vi "Tell Child.vi"(4 "Priority":bool, 6 "UID":string, 7 "Actor in":refnum<class "Actor.lvclass">, 9 "Error":errorcluster, 10 "Actor":refnum<class "Actor.lvclass">) -> (0 "Error out":errorcluster)   [LabVIEW 2025, in "jettl.lvlib" / "Stopped jettl Msg.lvlib"]
uses:
  Stopped jettl Msg.lvlib
  Actor/Actor.lvclass
  Msg Input/Msg Input.lvclass
  Stopped Msg/Stopped Msg/Stopped Msg.lvclass
  C:/git/jettl/src/jettl/jettl/Stopped jettl Msg/Stopped Msg/Stopped Msg/Stopped Msg.lvclass
  C:/git/jettl/src/jettl/jettl/Msg/Msg.lvclass
  jettl.lvlib
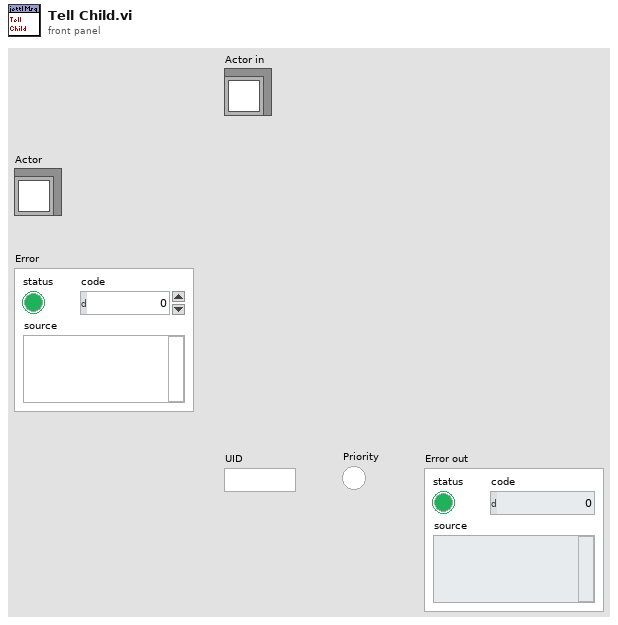
[diagram p1: front panel]
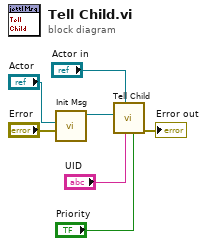
[diagram p0: block diagram]
diagram:
  n1 = call "Init Msg.vi"(9:"Error", "Msg Input"="Actor") -> ("Stopped Msg out"=w4:refnum<class "Stopped Msg.lvclass">)  [unwired: 9 in]
  n2 = call "Tell Child.vi"("Priority"="Priority", "UID"="UID", "Actor in"="Actor in", "Msg"=w4) -> ("Error out"=→"Error out":errorcluster)  [unwired: 7 in]
